vi "GetRightClickMenu.vi"(0 "reference":refnum<class "ClassDiagramGraph.lvclass">, 5 "error in (no error)":errorcluster) -> (14 "reference out":refnum<class "ClassDiagramGraph.lvclass">, 15 "Array":string[](array[string]), 16 "Found":bool, 19 "error out":errorcluster)   [LabVIEW 2016, in "ClassDiagramGraph.lvclass"]
uses:
  <resource>/Framework/Providers/Open_GDS/UML/ClassDiagramGraph_class/ClassDiagramGraph.lvclass
  C:/Program Files (x86)/National Instruments/LabVIEW 2016/resource/Framework/Providers/Open_GDS/UML/Graph_class/Graph.lvclass
  <resource>/Framework/Providers/Open_GDS/UML/ClassNode_class/ClassNode.lvclass
  <resource>/Framework/Providers/Open_GDS/UML/AbstractNode_class/AbstractNode.lvclass
  <resource>/Framework/Providers/Open_GDS/UML/Graph_class/Graph.lvclass
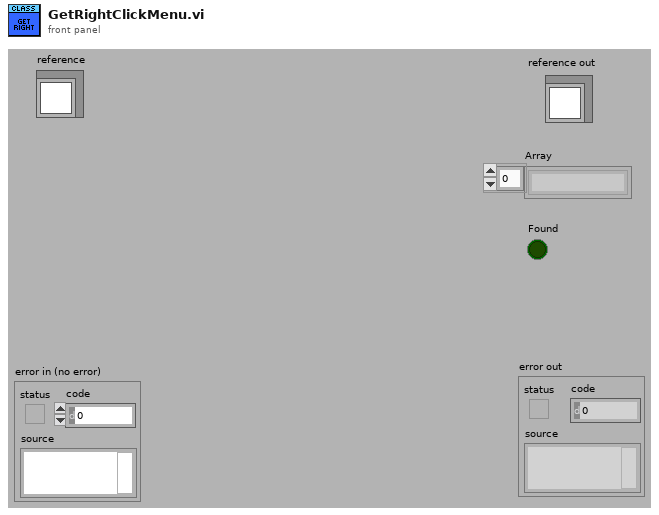
[diagram p1: front panel]
types:
  T1 = typedef "Graph.lvclass/ObjectAttributes.ctl" = cluster{"nodes":refnum<class "AbstractNode.lvclass">[], "edges":refnum<class "AbstractEdge.lvclass">[], "nodesToBeRemoved":refnum<class "AbstractNode.lvclass">[], "edgesToBeRemoved":refnum<class "AbstractEdge.lvclass">[], "needsLayout":bool, "LayoutNodes":refnum<class "AbstractNode.lvclass">[]}
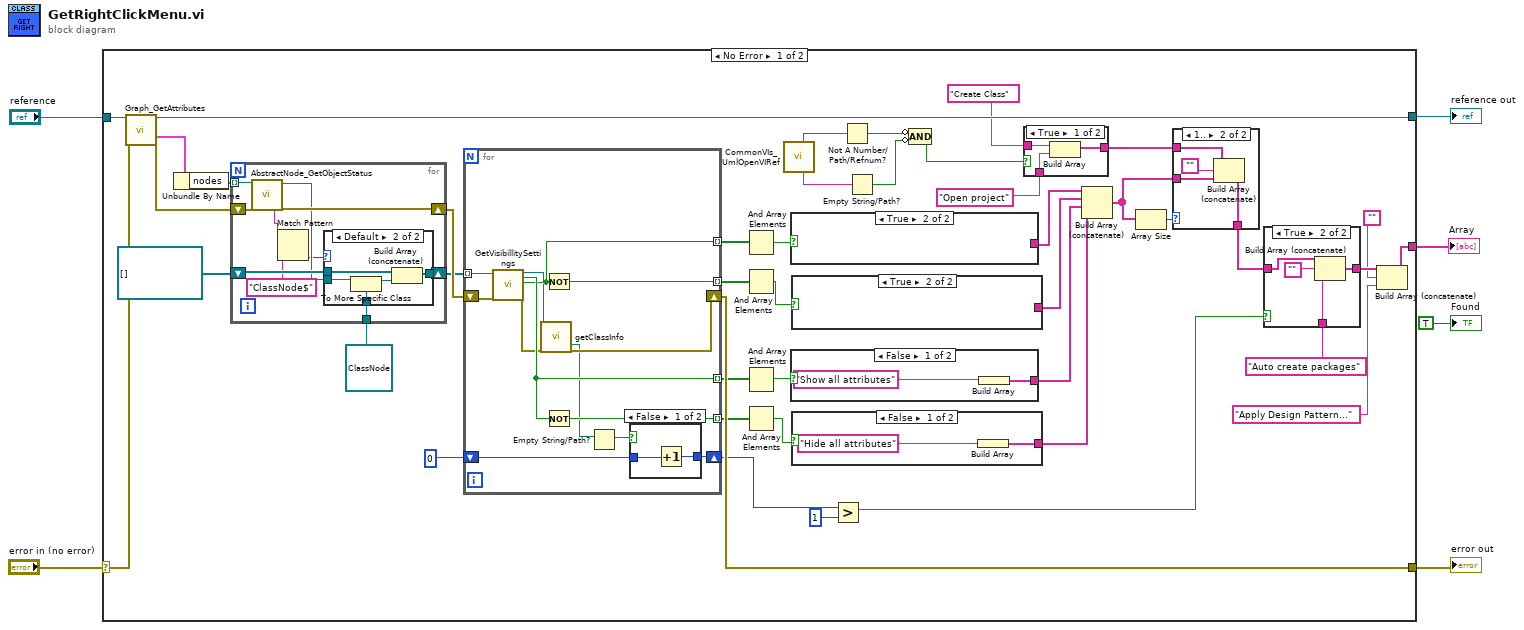
[diagram p0: block diagram]
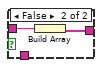
[diagram p3: hidden frame]
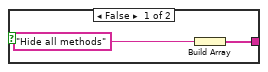
[diagram p7: hidden frame]
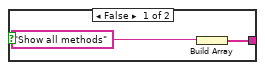
[diagram p8: hidden frame]
diagram:
  n1 = case shown="No Error" "error in (no error)" {
    selector: "error in (no error)" -> [w49 w105]
    tunnel: "reference" -> [w48 w106]
    tunnel: [w43 w105] -> w4
    tunnel: [w47 w106] -> w3
    tunnel: [w10 _] -> w2
    frame No Error {
      n2 = call <resource>:"Graph_GetAttributes.vi"("reference in"=w48, "error in (no error)"=w49) -> ("reference out"=w47:refnum<class "ClassDiagramGraph.lvclass">, "Data"=w7:T1, "error out"=w44:errorcluster)  [unwired: 14 in, 1 out]
      n3 = Unbundle By Name(w7) -> ("nodes"=w19:refnum<class "AbstractNode.lvclass">[])
      n4 = for {
        shift-right: [w96] -> w45
        shift-left: w44 -> [w98]
        tunnel: w19 -> [w97] mode=indexing
        shift-right: [w93] -> w17
        shift-left: refnum<class "ClassNode.lvclass">[] [] -> [w95]
        tunnel: refnum<class "ClassNode.lvclass"> refnum ("reference out") -> [w90]
        n5 = call <resource>:"AbstractNode_GetObjectStatus.vi"("reference in"=w97, "error in (no error)"=w98) -> ("Class name"=w89:string, "reference out"=w94:refnum<class "AbstractNode.lvclass">, "error out"=w96:errorcluster)  [unwired: 15 out]
        n6 = Match Pattern(string=w89, regular expression="ClassNode$") -> (offset past match=w91:i32)  [unwired: 4 out]
        n7 = case shown="Default" w91 {
          tunnel: w95 -> [w99 w104]
          tunnel: w94 -> [_ w102]
          tunnel: [w99 w103] -> w93
          tunnel: w90 -> [_ w100]
          frame -1 {
          }
          frame Default {
            n8 = To More Specific Class(target class=w100, reference=w102) -> (specific class reference=w101:refnum<class "ClassNode.lvclass">)  [unwired: 1 in, 1 out]
            n9 = Build Array (concatenate)(w104, w101) -> (w103:refnum<class "ClassNode.lvclass">[])
          }
        }
      }
      n10 = for {
        tunnel: w17 -> [w85] mode=indexing
        shift-right: [w78] -> w43
        shift-left: w45 -> [w84]
        tunnel: [w81] -> w39 mode=indexing
        tunnel: [w80] -> w40 mode=indexing
        tunnel: [w82] -> w34 mode=indexing
        tunnel: [w83] -> w33 mode=indexing
        shift-right: [w73] -> w15
        shift-left: 0 ("y") -> [w74]
        n11 = call <resource>:"GetVisibillitySettings.vi"("reference"=w85, "error in (no error)"=w84) -> ("reference out"=w76:refnum<class "ClassNode.lvclass">, "showAttribute"=w83:bool, "showMethods"=w80:bool, "error out"=w79:errorcluster)  [unwired: 14 out]
        n12 = call-dynamic "getClassInfo.vi"("reference"=w76, "error in (no error)"=w79) -> ("ClassPath"=w77:path, "error out"=w78:errorcluster)  [unwired: 8 in, 8 out]
        n13 = Not(x=w80) -> (.not. x?=w81:bool)
        n14 = Not(x=w83) -> (.not. x?=w82:bool)
        n15 = Empty String/Path?(string/path=w77) -> (empty?=w75:bool)
        n16 = case shown="False" w75 {
          tunnel: w74 -> [w87 w88]
          tunnel: [w86 w88] -> w73
          frame False {
            n17 = Increment(x=w87) -> (x+1=w86:i32)
          }
          frame True {
          }
        }
      }
      n18 = And Array Elements(Boolean array=w40) -> (logical AND=w38:bool)
      n19 = And Array Elements(Boolean array=w39) -> (logical AND=w37:bool)
      n20 = And Array Elements(Boolean array=w33) -> (logical AND=w32:bool)
      n21 = And Array Elements(Boolean array=w34) -> (logical AND=w31:bool)
      n22 = call <resource>:"CommonVIs_UmlOpenVIRef.vi"() -> ("ProjectNameOut"=w25:string, "AppRefOut"=w26:refnum<vi>)  [unwired: 4 in, 6 out]
      n23 = case shown="True" w38 {
        tunnel: [w72 _] -> w42
        frame False {
          n24 = Build Array("Show all methods") -> (w72:string[])
        }
        frame True {
        }
      }
      n25 = case shown="False" w32 {
        tunnel: [w63 _] -> w30
        frame False {
          n26 = Build Array("Show all attributes") -> (w63:string[])
        }
        frame True {
        }
      }
      n27 = case shown="True" w37 {
        tunnel: [w70 _] -> w41
        frame False {
          n28 = Build Array("Hide all methods") -> (w70:string[])
        }
        frame True {
        }
      }
      n29 = case shown="False" w31 {
        tunnel: [w61 _] -> w29
        frame False {
          n30 = Build Array("Hide all attributes") -> (w61:string[])
        }
        frame True {
        }
      }
      n31 = Greater?(x=w15, y=1) -> (0:w13:bool)
      n32 = Not A Number/Path/Refnum?(number/path/refnum=w26) -> (NaN/Path/Refnum?=w24:bool)
      n33 = Empty String/Path?(string/path=w25) -> (empty?=w23:bool)
      n34 = Compound Arithmetic op=AND(invert w24, invert w23) -> (w22:bool)
      n35 = case shown="True" w22 {
        tunnel: "Create Class" -> [w57 w59]
        tunnel: [w56 w58] -> w27
        tunnel: "Open project" ("element") -> [w55 _]
        frame True {
          n36 = Build Array(w57, w55) -> (w56:string[])
        }
        frame False {
          n37 = Build Array(w59) -> (w58:string[])
        }
      }
      n38 = Build Array (concatenate)(w42, w41, w30, w29) -> (w36:string[])
      n39 = Array Size(array=w36) -> (size(s)=w35:i32)
      n40 = case shown="1.." w35 {
        tunnel: [w64 w68] -> w14
        tunnel: w27 -> [w64 w67]
        tunnel: w36 -> [_ w66]
        frame Default {
        }
        frame 1.. {
          n41 = Build Array (concatenate)(w67, "", w66) -> (w68:string[])
        }
      }
      n42 = case shown="True" w13 {
        tunnel: w14 -> [w50 w52]
        tunnel: [w50 w53] -> w11
        tunnel: "Auto create packages" -> [_ w51]
        frame False {
        }
        frame True {
          n43 = Build Array (concatenate)(w52, "", w51) -> (w53:string[])
        }
      }
      n44 = Build Array (concatenate)(w11, "", "Apply Design Pattern..." ("element")) -> (w10:string[])
    }
    frame Error {
    }
  }
  "reference out" <- w3
  "error out" <- w4
  "Array" <- w2
  "Found" <- TRUE ("Found")
